vi "GetHelp.vi"(11 "VIPMInstallPackageFile in":refnum<class "VIPMInstallPackageFile.lvclass">) -> (2 "Help":string, 3 "VIPMInstallPackageFile out":refnum<class "VIPMInstallPackageFile.lvclass">)   [LabVIEW 2014, in "VIPMInstallPackageFile.lvclass"]
uses:
  <nishared>/LabVIEW CLI/Operations/VIPMInstallPackageFile/VIPMInstallPackageFile.lvclass
panel:
  in  "Help":string="LabVIEWCLI -OperationName VIPMInstallPackageFile -PackagePath <path of VIPM package file (.vip)> -LabVIEWVersion <labview version string>\n\n -PackagePath : Specifies the path to the VIPM package file (.vip) to install\n\n -LabVIEWVersion : Specifies the version of LabVIEW to install the VIPM package to (e.g. \"17.0\", \"17.0 (64-bit)\", \"18.0\", \"18.0 (64-bit)\", ...)\n\nNote: You must have the VIPM API installed and have a JKI VI Package Manager Pro license.\n"
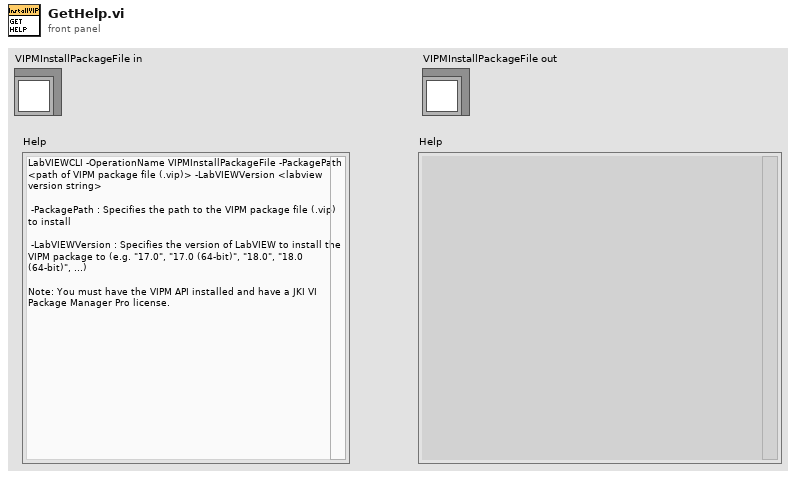
[diagram p1: front panel]
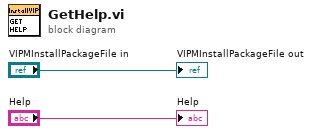
[diagram p0: block diagram]
diagram:
  "VIPMInstallPackageFile out" <- "VIPMInstallPackageFile in"
  "Help" <- "Help"
